vi "Get GObj General Properties(冲突时的文件备份2013-05-03 10-29-29).vi"(8 "错误输入（无错误）":errorcluster, 11 "GObj Ref In":refnum<vi>) -> (0 "错误输出":errorcluster, 2 "General Property":T1, 3 "GObj Ref Out":refnum<vi>)   [LabVIEW 2012, in "CtrlRef.lvlib"]
uses:
  CtrlRef.lvlib
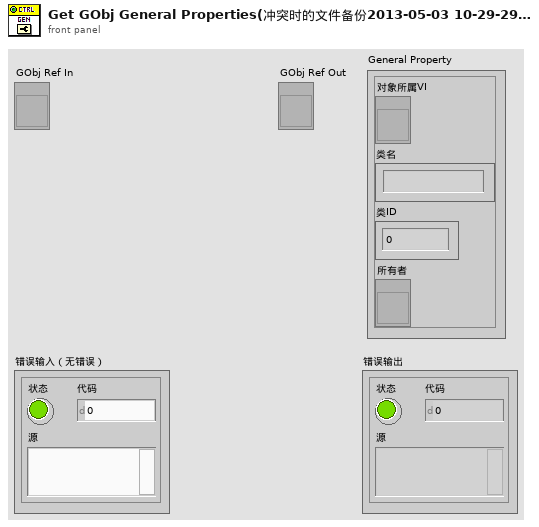
[diagram p1: front panel]
types:
  T1 = cluster{"对象所属VI":refnum<vi>, "类名":string, "类ID":u32, "所有者":refnum<vi>}
  T2 = cluster{"OwningVI":refnum<vi>, "ClassName":string, "ClassID":u32, "Owner":refnum<vi>}
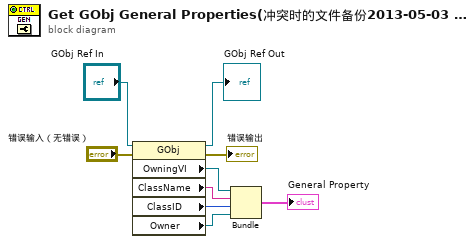
[diagram p0: block diagram]
diagram:
  n1 = property class="GObj"(reference="GObj Ref In", error in="错误输入（无错误）") -> (reference out=→"GObj Ref Out":refnum<vi>, error out=→"错误输出":errorcluster, "OwningVI"=w7:refnum<vi>, "ClassName"=w6:string, "ClassID"=w5:u32, "Owner"=w4:refnum<vi>)
  n2 = Bundle("OwningVI"=w7, "ClassName"=w6, "ClassID"=w5, "Owner"=w4) -> (→"General Property":T2)  [unwired: 1 in]
